vi "Upload to Arduino.vi"() -> ()   [LabVIEW 2020]
panel:
  in  "code":string="/*\n  Blink\n\n  Turns an LED on for one second, then off for one second, repeatedly.\n\n  Most Arduinos have an on-board LED you can control. On the UNO, MEGA and ZERO\n  it is attached to digital pin 13, on MKR1000 on pin 6. LED_BUILTIN is set to\n  the correct LED pin independent of which board is used.\n  If you want to know what pin the on-board LED is connected to on your Arduino\n  model, check the Technical Specs of your board at:\n  https://www.arduino.cc/en/Main/Products\n\n  modified 8 May 2014\n  by Scott Fitzgerald\n  modified 2 Sep 2016\n  by Arturo Guadalupi\n  modified 8 Sep 2016\n  by Colby Newman\n\n  This example code is in the public domain.\n\n  http://www.arduino.cc/en/Tutorial/Blink\n*/\n\n// the setup function runs once when you press reset or power the board\nvoid setup() {\n  // initialize digital pin LED_BUILTIN as an output.\n  pinMode(LED_BUILTIN, OUTPUT);\n}\n\n// the loop function runs over and over again forever\nvoid loop() {\n  digitalWrite(LED_BUILTIN, HIGH);   // turn the LED on (HIGH is the voltage level)\n  delay(2000);                       // wait for a second\n  digitalWrite(LED_BUILTIN, LOW);    // turn the LED off by making the voltage LOW\n  delay(2000);                       // wait for a second\n}"
  out "Output":string="***** Complie *****\nSketch uses 11292 bytes (4%) of program storage space. Maximum is 262144 bytes.\n\n\n***** Set Baud *****\n\n\n***** Upload *****\nSet binary mode\nreadWord(addr=0)=0x20007ffc\nreadWord(addr=0xe000ed00)=0x410cc601\nreadWord(addr=0x41002018)=0x10010305\nversion()=v2.0 [Arduino:XYZ] Apr 19 2019 14:38:48\nchipId=0x10010005\nConnected at 921600 baud\nreadWord(addr=0)=0x20007ffc\nreadWord(addr=0xe000ed00)=0x410cc601\nreadWord(addr=0x41002018)=0x10010305\nAtmel SMART device 0x10010005 found\nwrite(addr=0x20004000,size=0x34)\nwriteWord(addr=0x20004030,value=0x10)\nwriteWord(addr=0x20004020,value=0x20008000)\nDevice       : ATSAMD21G18A\nreadWord(addr=0)=0x20007ffc\nreadWord(addr=0xe000ed00)=0x410cc601\nreadWord(addr=0x41002018)=0x10010305\nChip ID      : 10010005\nversion()=v2.0 [Arduino:XYZ] Apr 19 2019 14:38:48\nVersion      : v2.0 [Arduino:XYZ] Apr 19 2019 14:38:48\nAddress      : 8192\nPages        : 3968\nPage Size    : 64 bytes\nTotal Size   : 248KB\nPlanes       : 1\nLock Regions : 16\nLocked       : readWord(addr=0x41004020)=0xffff\nreadWord(addr=0x41004020)=0xffff\nreadWord(addr=0x41004020)=0xffff\nreadWord(addr=0x41004020)=0xffff\nreadWord(addr=0x41004020)=0xffff\nreadWord(addr=0x41004020)=0xffff\nreadWord(addr=0x41004020)=0xffff\nreadWord(addr=0x41004020)=0xffff\nreadWord(addr=0x41004020)=0xffff\nreadWord(addr=0x41004020)=0xffff\nreadWord(addr=0x41004020)=0xffff\nreadWord(addr=0x41004020)=0xffff\nreadWord(addr=0x41004020)=0xffff\nreadWord(addr=0x41004020)=0xffff\nreadWord(addr=0x41004020)=0xffff\nreadWord(addr=0x41004020)=0xffff\nnone\nreadWord(addr=0x41004018)=0\nSecurity     : false\nBoot Flash   : true\nreadWord(addr=0x40000834)=0x7000a\nBOD          : true\nreadWord(addr=0x40000834)=0x7000a\nBOR          : true\nArduino      : FAST_CHIP_ERASE\nArduino      : FAST_MULTI_PAGE_WRITE\nArduino      : CAN_CHECKSUM_MEMORY_BUFFER\nErase flash\nchipErase(addr=0x2000)\ndone in 0.824 seconds\n\nWrite 11436 bytes to flash (179 pages)\nwrite(addr=0x20005000,size=0x1000)\nwriteBuffer(scr_addr=0x20005000, dst_addr=0x2000, size=0x1000)\n\r[==========                    ] 35% (64/179 pages)write(addr=0x20005000,size=0x1000)\nwriteBuffer(scr_addr=0x20005000, dst_addr=0x3000, size=0x1000)\n\r[=====================         ] 71% (128/179 pages)write(addr=0x20005000,size=0xcc0)\nwriteBuffer(scr_addr=0x20005000, dst_addr=0x4000, size=0xcc0)\n\r[==============================] 100% (179/179 pages)\ndone in 0.077 seconds\n\nVerify 11436 bytes of flash with checksum.\nchecksumBuffer(start_addr=0x2000, size=0x1000) = 6bed\nchecksumBuffer(start_addr=0x3000, size=0x1000) = cf07\nchecksumBuffer(start_addr=0x4000, size=0xcac) = 8e51\nVerify successful\ndone in 0.010 seconds\nCPU reset.\nreadWord(addr=0)=0x20007ffc\nreadWord(addr=0xe000ed00)=0x410cc601\nreadWord(addr=0x41002018)=0x10010305\nwriteWord(addr=0xe000ed0c,value=0x5fa0004)\n\n\n"
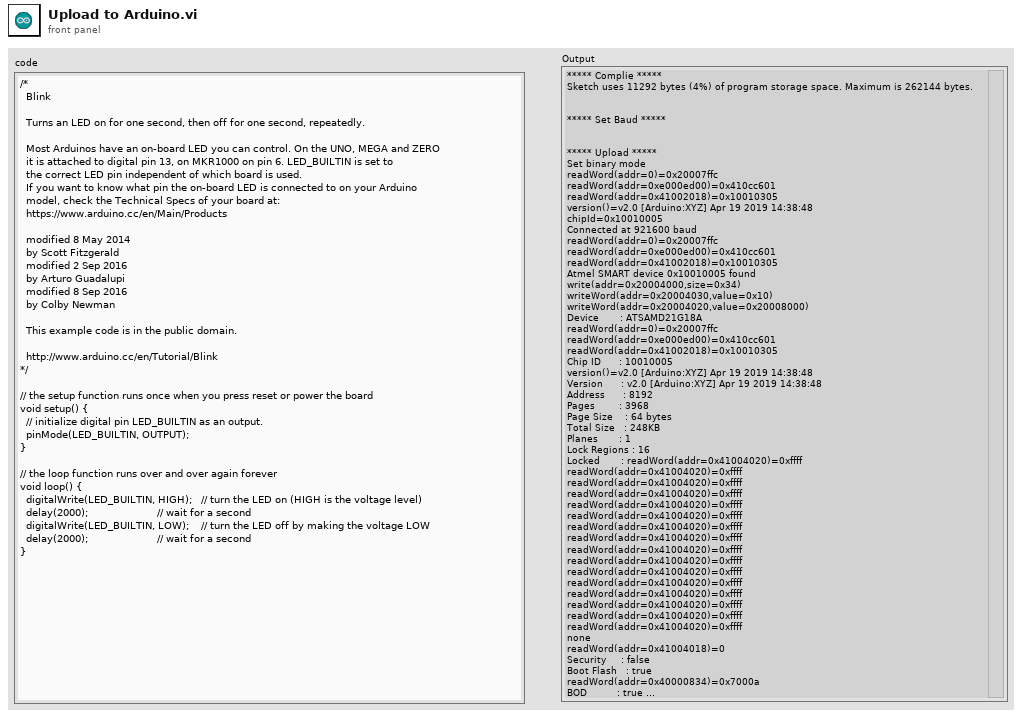
[diagram p1: front panel]
types:
  T1 = typedef "Arduino.ctl" = cluster{"Java":path, "Packages":path, "folder":path, "serial":string, "Console":string}
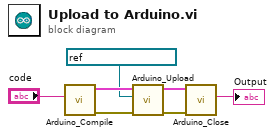
[diagram p0: block diagram]
diagram:
  n1 = call "Arduino_Compile.vi"("Code"="code") -> ("error out"=w7:errorcluster, "Arduino Out"=w5:T1)  [unwired: 9 in]
  n2 = call "Arduino_Upload.vi"("error in (no error)"=w7, "VISA resource name"=refnum<visa-resource-name> "ASRL22::INSTR" ("VISA"), "Arduino In"=w5) -> ("error out"=w6:errorcluster, "Arduino Out"=w4:T1)  [unwired: 7 in]
  n3 = call "Arduino_Close.vi"("error in (no error)"=w6, "Arduino In"=w4) -> ("Console"=→"Output":string)  [unwired: 8 in, 1 out]
